vi "TAT_Start.vi"(8 "error In":errorcluster) -> (0 "error out":errorcluster)   [LabVIEW 2017]
uses:
  <vilib>/Utility/error.llb/DialogType.ctl
  Controls/Ass. Loop Control.ctl
  <vilib>/addons/database/Connection.llb/Conn ObjectReference.ctl
  227c0874-5cf7-40bb-b9d2-311cfb67fe7f.vi
  Global/Global 1.vi
  <vilib>/Instr/_visa.llb/VISA Configure Serial Port (Instr).vi
  <vilib>/addons/database/NI_Database_API.lvlib
  <vilib>/Utility/config.llb/NI_LVConfig.lvlib
panel:
  in  "MODEL SELECTION:-":string(combo)
  out "12 4":bool
  out "EOL AUTO CYCLE STATUS:-":bool
  out "12 3":bool
  out "12 2":bool
  out "12":bool
  out "PLC STATUS:-":bool
  out "array":string[](array[string])
  out "LEAK UNIT RESULT 2":bool caption="LEAK RESULT:-"
  out "LEAK ACTUAL VALUE 2":string
  out "LEAK MAX 2":string
  out "LEAK MIN 2":string
  out "LEAK UNIT RESULT":bool caption="LEAK RESULT:-"
  out "LEAK ACTUAL VALUE":string
  out "LEAK MAX":string
  out "LEAK MIN":string
  out "PREVIOUS BARCODE":string[](array[string])
  out "scanned":string
  out "Scanned Qyt":string
  out "PROJECT :-":string
  out "PACKAGE Qty":string
  out "TORISHI CODE:-":string
  out "PART No.:-":string
  in  "Stop":bool
  out "BARCODE STATION 2":string caption="BARCODE:-"
  out "RESULT STATION 1":bool caption="FINAL RESULT:-"
  out "USER:-":string
  out "PART NAME :-":string
  in  "ASS-Alarms":bool
  out "CYCLE STATUS STATION 1":string caption="CYCLE STATUS:-"
  out "DATE/TIME":string
  # "KAPSE SONS ROBOTICS\n& AUTOMATION"
  # "Nm"
  # "POKA-YOKE STATUS"
  # "LEAK TESTING PARAMETER"
  # "MIN"
  # "MAX"
  # "ACTUAL VALUE"
  # "RESULT"
  # "LEAK UNIT"
  # "LEAK PRESSURE"
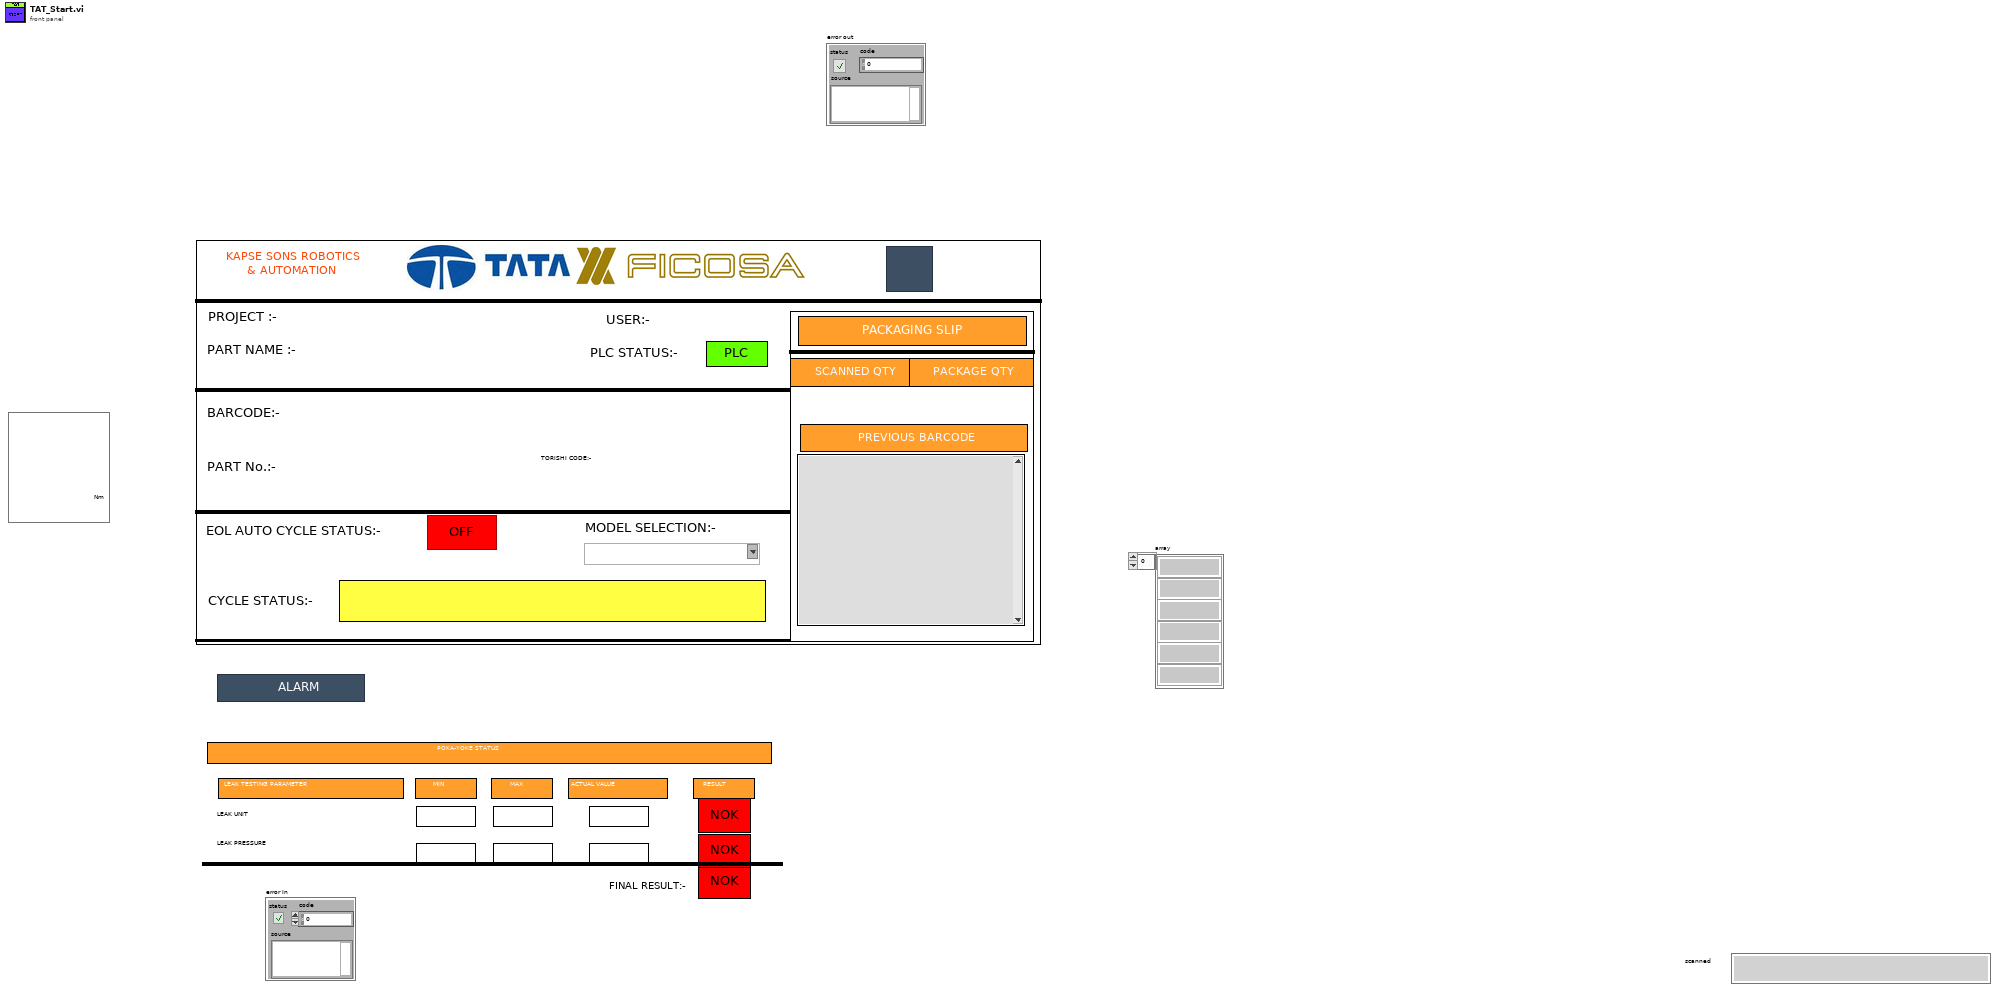
[diagram p1: front panel]
types:
  T1 = typedef "NI_Database_API.lvlib/Conn ObjectReference.ctl" = refnum<k1>
  T2 = cluster{"Varient number":u16, "Part name":string, "Barcode":string, "connection reference":T1, "Batch_Size":u16, "PART_NO":string, "TORISHI_CODE":string, "scanner com":refnum<visa-resource-name>, "Part Name List":string[], "Varient path":path, "Current Varient path":path, "Communication path":path, "PRN path":path, "printer":refnum<k5>, "Data_log_Path":path, "PREVIOUS Code":string[], "Printer IP add":string}
  T3 = typedef "Ass. Loop Control.ctl" = enum16{"Int2", "Package_Qty_Count", "GENERATE_QR_PRNT", "Cluster_update", "Waiting_for_scan", "barcode CHECK", "Int", "SaveReport ", "Barcode Print", "Start Cycle", "Wait", "Cycle End", "Stop"}
  T4 = typedef "DialogType.ctl" = u16
  T5 = enum32{"invalid app kind", "Development System", "Run Time System", "Student Edition", "Embedded LabVIEW", "Evaluation", "Custom"}
  T6 = typedef "NI_LVConfig.lvlib/Config Data RefNum.ctl" = refnum<k1>
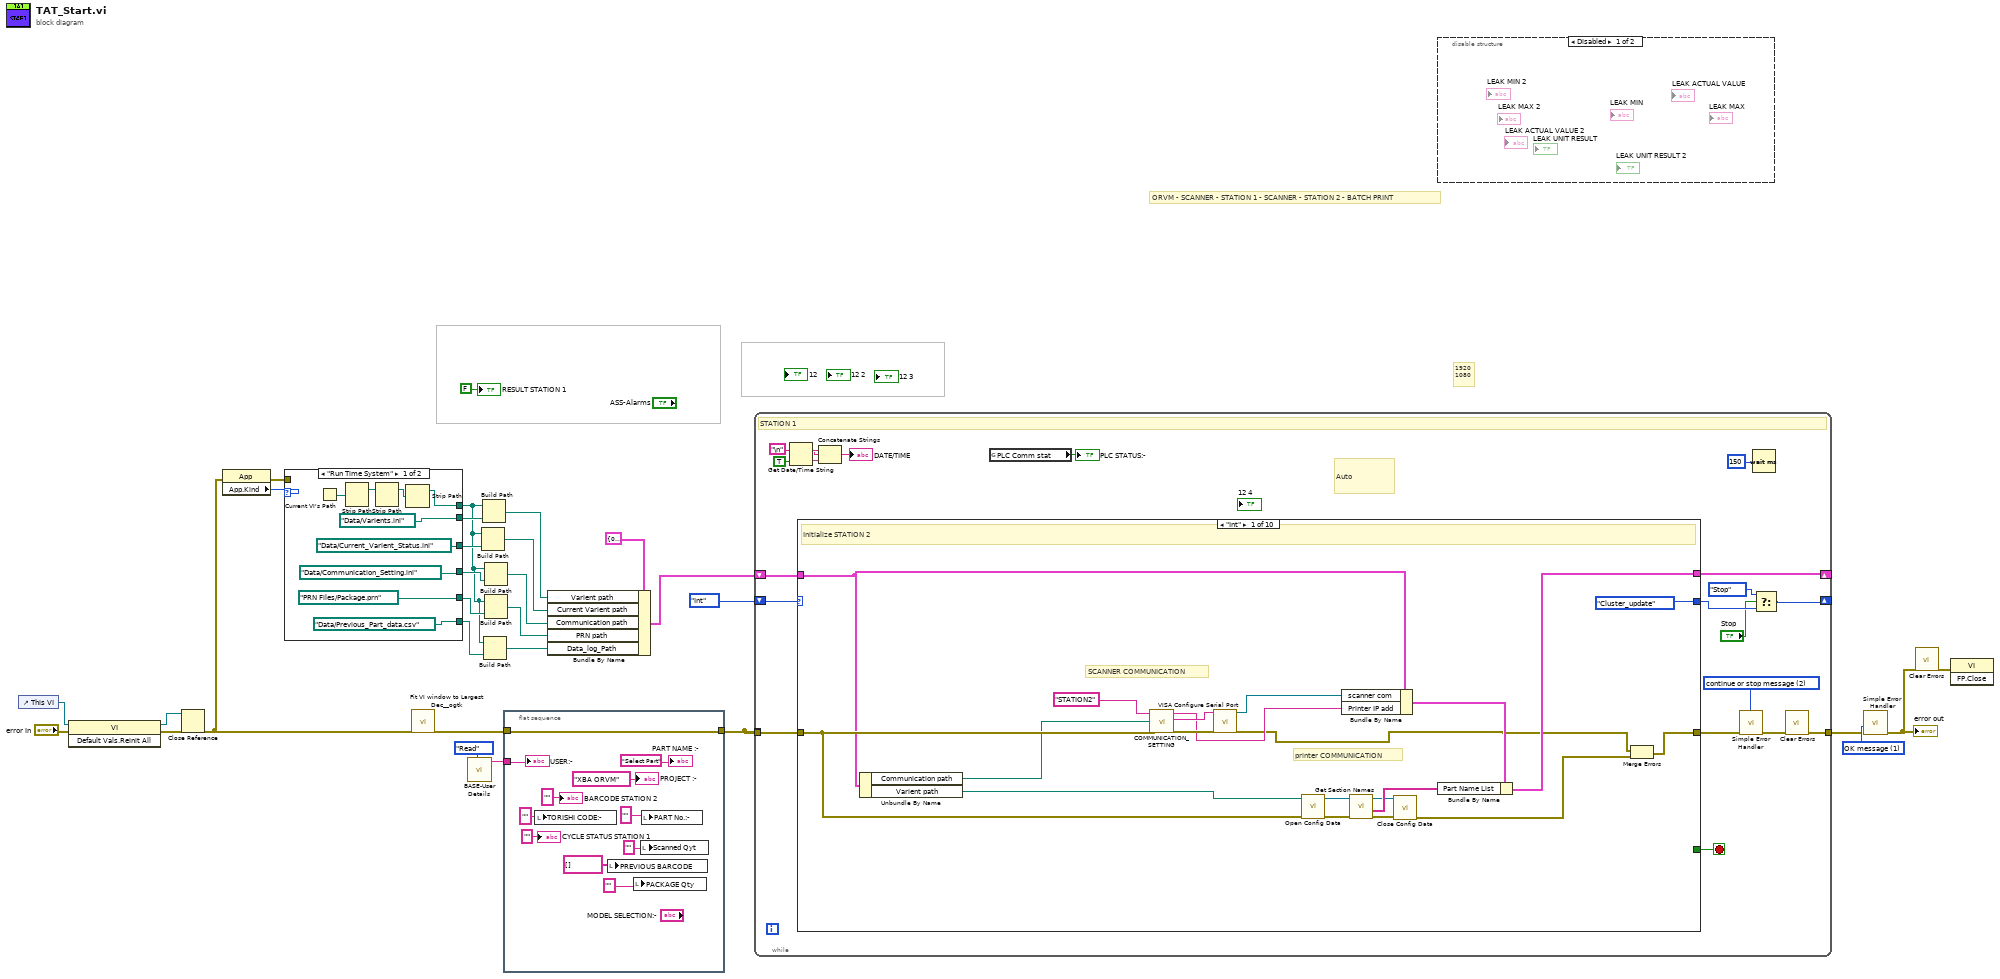
[diagram p0: block diagram]
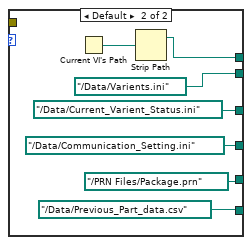
[diagram p2: hidden frame]
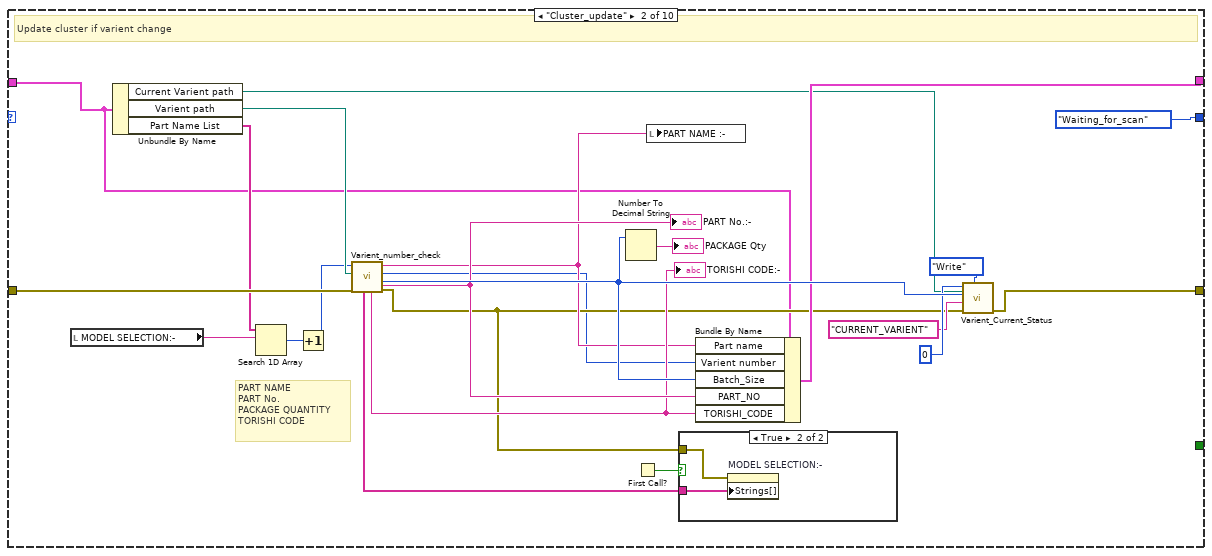
[diagram p4: hidden frame]
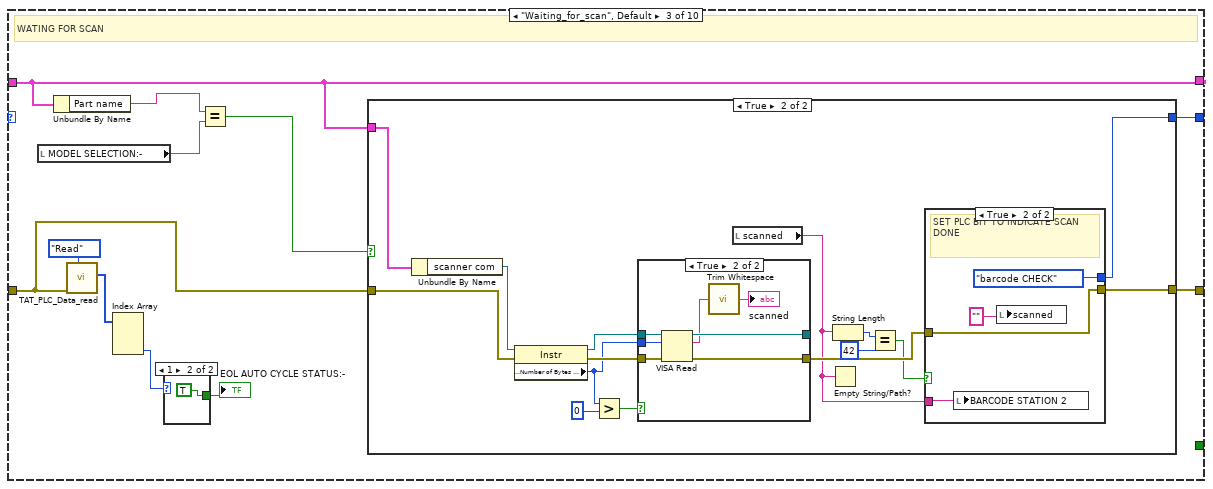
[diagram p6: hidden frame]
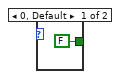
[diagram p7: hidden frame]
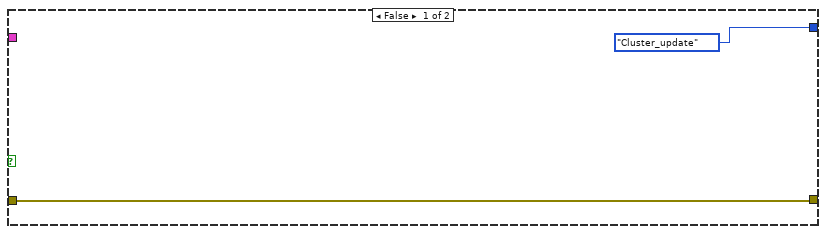
[diagram p8: hidden frame]
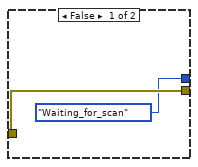
[diagram p10: hidden frame]
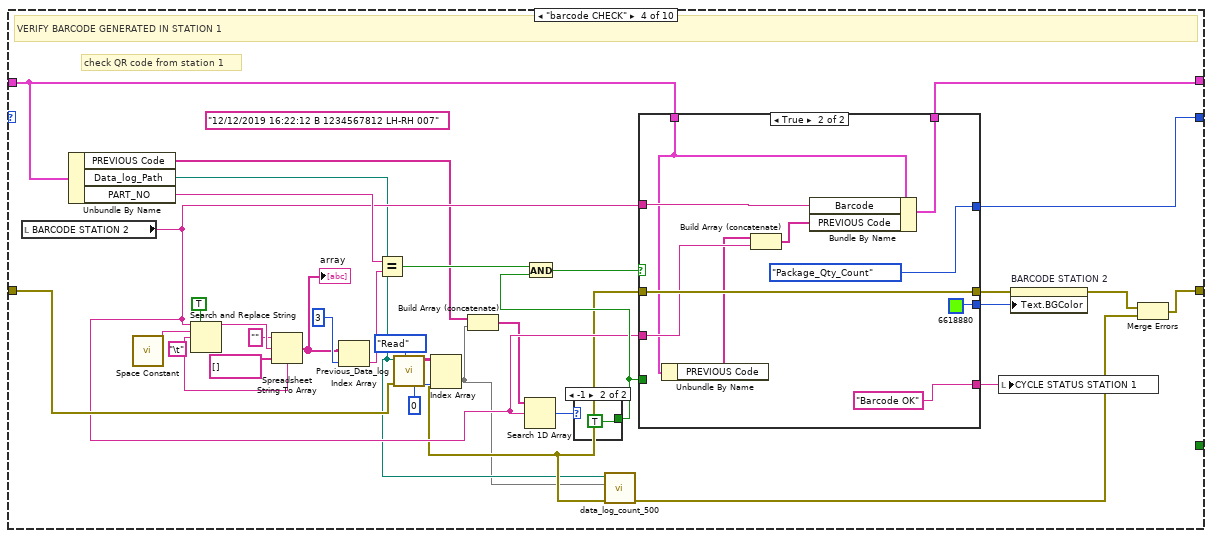
[diagram p11: hidden frame]
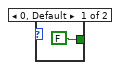
[diagram p12: hidden frame]
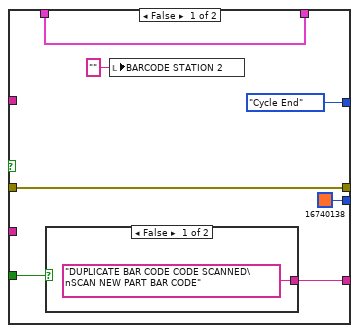
[diagram p13: hidden frame]
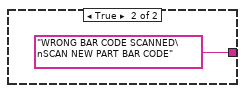
[diagram p14: hidden frame]
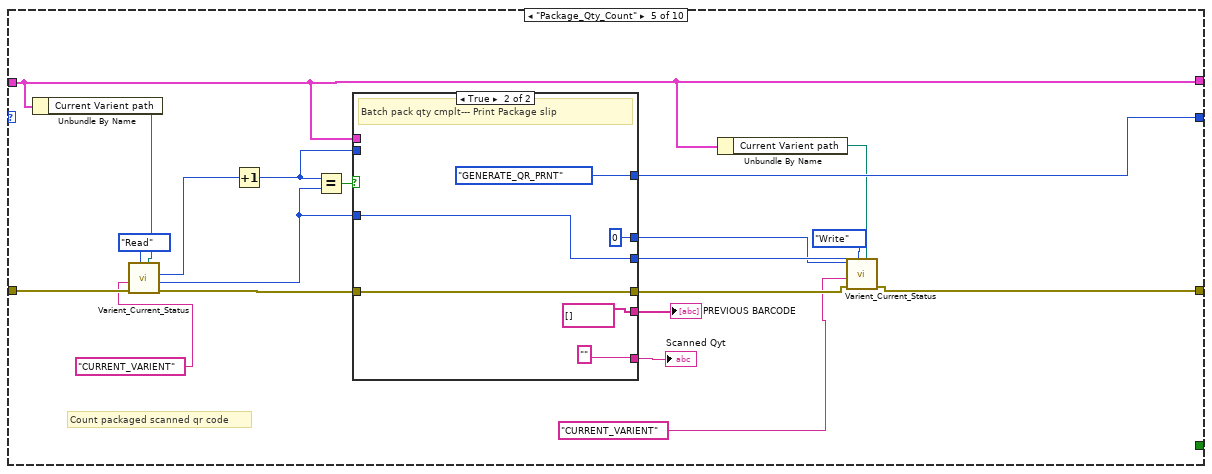
[diagram p15: hidden frame]
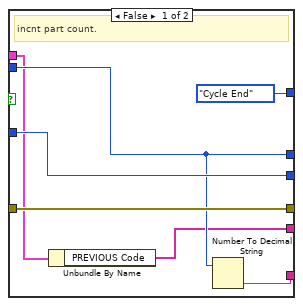
[diagram p16: hidden frame]
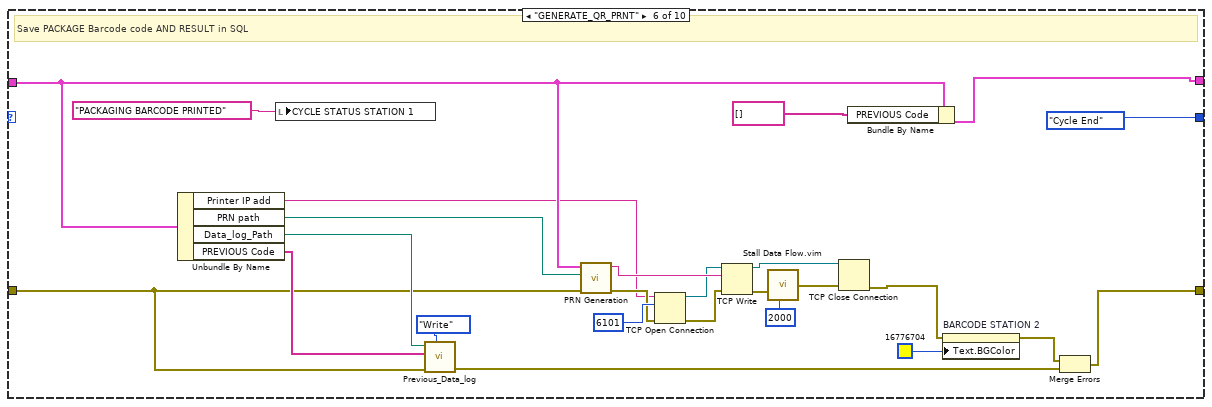
[diagram p17: hidden frame]
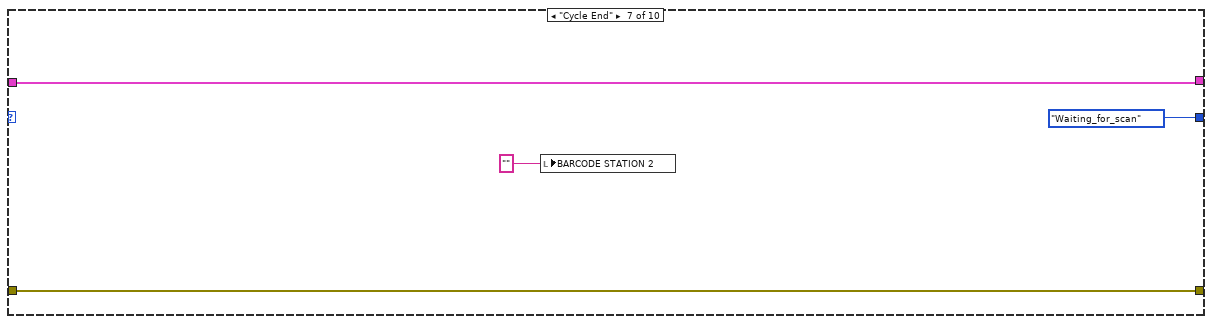
[diagram p18: hidden frame]
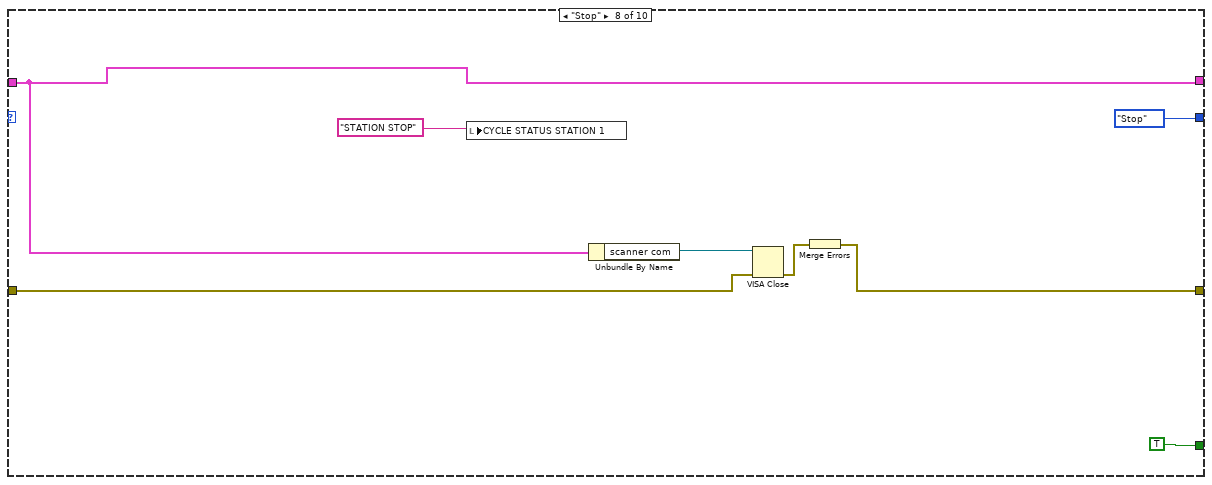
[diagram p19: hidden frame]
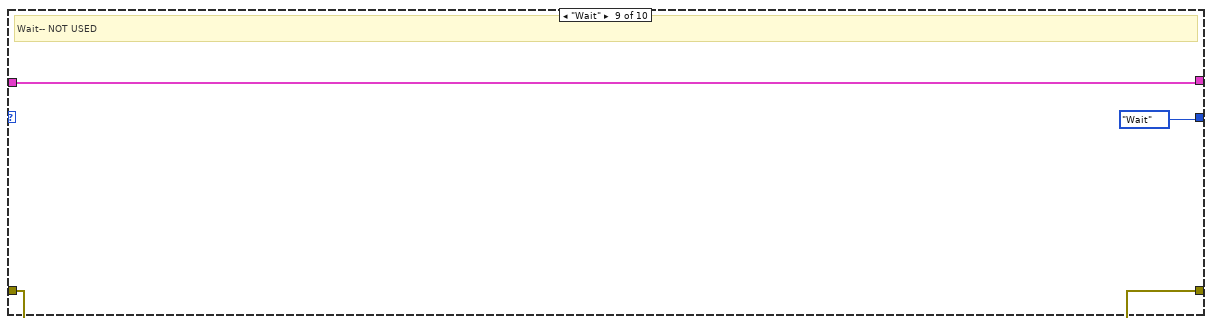
[diagram p20: hidden frame]
diagram:
  w20 = T4 1 items=["no dialog", "OK message", "continue or stop message", "OK message + warnings", "continue/stop + warnings"] ("type of dialog (OK msg:1)")
  # "1920\n1080"
  # "ORVM - SCANNER - STATION 1 - SCANNER - STATION 2 - BATCH PRINT"
  n1 = control-ref of="This VI"() -> (w30:refnum<vi>)
  n2 = invoke class="VI" method="Default Vals.Reinit All"(reference=w30, error in="error In") -> (reference out=w27:refnum<vi>, error out=w28:errorcluster)  [unwired: 1 in, 1 out]
  n3 = Close Reference(reference=w27, error in (no error)=w28) -> (error out=w4:errorcluster)
  n4 = property class="App"(error in=w4) -> (error out=w7:errorcluster, "App.Kind"=w16:T5)  [unwired: 1 in, 1 out]
  n5 = case shown="\"Run Time System\"" w16 {
    tunnel: [path "Data/Varients.ini" ("path") path "../Data/Varients.ini" ("path")] -> w15
    tunnel: [w35 w44] -> w5
    tunnel: [path "Data/Current_Varient_Status.ini" ("path") path "../Data/Current_Varient_Status.ini" ("path")] -> w12
    tunnel: [path "Data/Communication_Setting.ini" ("path") path "../Data/Communication_Setting.ini" ("path")] -> w11
    tunnel: [path "PRN Files/Package.prn" ("path") path "../PRN Files/Package.prn" ("path")] -> w9
    tunnel: w7 -> [_ _]
    tunnel: [path "Data/Previous_Part_data.csv" ("path") path "../Data/Previous_Part_data.csv" ("path")] -> w1
    frame "Run Time System" {
      n6 = Current VI's Path() -> (path=w38:path)
      n7 = Strip Path(path=w38) -> (stripped path=w37:path)  [unwired: 1 out]
      n8 = Strip Path(path=w37) -> (stripped path=w36:path)  [unwired: 1 out]
      n9 = Strip Path(path=w36) -> (stripped path=w35:path)  [unwired: 1 out]
    }
    frame Default {
      n10 = Current VI's Path() -> (path=w45:path)
      n11 = Strip Path(path=w45) -> (stripped path=w44:path)  [unwired: 1 out]
    }
  }
  n12 = call <userlib>:"Fit VI window to Largest Dec__ogtk.vi"("error in (no error)"=w4) -> ("error out"=w26:errorcluster)  [unwired: 5 in, 1 out]
  n13 = call "BASE-User Details.vi"("Enum"=enum16{"Read", "Write"}."Read") -> ("User Name Out"=w21:string)  [unwired: 9 in, 1 out]
  n14 = Build Path(base path=w5, name or relative path=w12) -> (appended path=w13:path)
  n15 = Build Path(base path=w5, name or relative path=w15) -> (appended path=w14:path)
  n16 = Build Path(base path=w5, name or relative path=w1) -> (appended path=w6:path)
  n17 = Build Path(base path=w5, name or relative path=w11) -> (appended path=w10:path)
  n18 = Build Path(base path=w5, name or relative path=w9) -> (appended path=w8:path)
  n19 = flat-sequence {
    tunnel: [w57] -> w18
    tunnel: w26 -> [w57]
    tunnel: w21 -> [w56]
    frame #0 {
      n20 = local write "TORISHI CODE:-"("") -> ()
      n21 = local write "PREVIOUS BARCODE"(string[] []) -> ()
      n22 = local write "PACKAGE Qty"("") -> ()
      n23 = local write "Scanned Qyt"("") -> ()
      n24 = local write "PART No.:-"("") -> ()
      "USER:-" <- w56
      "PART NAME :-" <- "Select Part"
      "PROJECT :-" <- "XBA ORVM" ("PROJECT")
      "BARCODE STATION 2" <- ""
      "CYCLE STATUS STATION 1" <- ""
    }
  }
  n25 = Bundle By Name(cluster=T2 {"Varient number"=0, "Part name"="", "Barcode"="", "connection reference"=refnum, "Batch_Size"=0, "PART_NO"="", "TORISHI_CODE"="", "scanner com"="", "Part Name List"=[], "Varient path"=path "", "Current Varient path"=path "", "Communication path"=path "", "PRN path"=path "", "printer"=refnum, "Data_log_Path"=path "", "PREVIOUS Code"=[], "Printer IP add"=""}, "Varient path"=w14, "Current Varient path"=w13, "Communication path"=w10, "PRN path"=w8, "Data_log_Path"=w6) -> (w2:T2)
  n26 = while {
    tunnel: w18 -> [_]
    shift-right: [w66] -> _
    shift-left: Ass._Loop_Control."Int" ("Enum") -> [w71]
    tunnel: w18 -> [w70]
    shift-right: [w68] -> _
    shift-left: w2 -> [w69]
    tunnel: [w59] -> w17
    stop <- w58 stop-if-true
    w63 = T4 2 items=["no dialog", "OK message", "continue or stop message", "OK message + warnings", "continue/stop + warnings"] ("type of dialog (OK msg:1)")
    # "Auto"
    # "STATION 1"
    n27 = Get Date/Time String(want seconds? (F)=TRUE) -> (date string=w75:string, time string=w74:string)  [unwired: 2 in]
    n28 = case shown="\"Int\"" w71 {
      tunnel: [Ass._Loop_Control."Cluster_update" ("Enum") Ass._Loop_Control."Waiting_for_scan" ("Enum") w132 w176 w230 Ass._Loop_Control."Cycle End" ("Enum") Ass._Loop_Control."Waiting_for_scan" ("Enum") Ass._Loop_Control."Stop" ("Enum") Ass._Loop_Control."Wait" ("Enum") Ass._Loop_Control."Wait" ("Enum")] -> w65
      tunnel: [w84 w112 w129 w198 w222 w274 w282 w287 w294 w295] -> w68
      tunnel: [w83 w113 w133 w173 w235 w266 w280 w288 w292 w296] -> w62
      tunnel: w70 -> [w93 w107 w123 w180 w241 w268 w280 w285 w292 w296]
      tunnel: w69 -> [w92 w98 w129 w199 w222 w263 w282 w287 w294 w295]
      tunnel: [_ _ _ _ _ _ _ TRUE _ _] -> w58
      frame "Int" {
        # "printer COMMUNICATION"
        # "SCANNER COMMUNICATION"
        # "Initialize STATION 2"
        n29 = Unbundle By Name(w92) -> ("Communication path"=w81:path, "Varient path"=w82:path)
        n30 = call "COMMUNICATION_SETTING.vi"("communication path"=w81, "error in"=w93, "STATION"="STATION2") -> ("error out"=w96:errorcluster, "SCAN_COM"=w94:string, "PRINT_COM"=w80:string)  [unwired: 6 in]
        n31 = call-poly "VISA Configure Serial Port"("VISA resource name"=w94, "error in (no error)"=w96) -> ("VISA resource name out"=w78:refnum<visa-resource-name>, "error out"=w79:errorcluster)  [unwired: 12 in]
        n32 = call <vilib>:"Open Config Data.vi"("error in (no error)"=w93, "configuration file path"=w82) -> ("error out"=w89:errorcluster, "refnum"=w90:T6)  [unwired: 7 in, 1 out]
        n33 = Bundle By Name(cluster=w92, "scanner com"=w78, "Printer IP add"=w80) -> (w85:T2)
        n34 = call <vilib>:"Get Section Names.vi"("error in (no error)"=w89, "refnum"=w90) -> ("error out"=w88:errorcluster, "section names"=w91:string[], "refnum out"=w87:T6)  [unwired: 7 in]
        n35 = call <vilib>:"Close Config Data.vi"("error in (no error)"=w88, "refnum"=w87) -> ("error out"=w86:errorcluster)  [unwired: 8 in, 1 out]
        n36 = Bundle By Name(cluster=w85, "Part Name List"=w91) -> (w84:T2)
        n37 = Merge Errors(w79, w86) -> (w83:errorcluster)
      }
      frame "Cluster_update" {
        # "PART NAME\nPART No.\nPACKAGE QUANTITY\nTORISHI CODE"
        # "Update cluster if varient change"
        n38 = local read "MODEL SELECTION:-"() -> (w101:string)
        n39 = Unbundle By Name(w98) -> ("Current Varient path"=w108:path, "Varient path"=w109:path, "Part Name List"=w102:string[])
        n40 = Search 1D Array(1D array=w102, element=w101) -> (index of element=w103:i32)  [unwired: 1 in]
        n41 = Increment(x=w103) -> (x+1=w100:i32)
        n42 = call "Varient_number_check.vi"("error in"=w107, "Varient path"=w109, "Varient No."=w100) -> ("error out"=w104:errorcluster, "Batch Size"=w120:i32, "Varient Number"=w99:i32, "Part Name"=w116:string, "PART_NO"=w119:string, "TORISHI_CODE"=w118:string, "MODEL LIST"=w105:string[])  [unwired: 2 in]
        "PART No.:-" <- w119
        "TORISHI CODE:-" <- w118
        n43 = Number To Decimal String(number=w120) -> (decimal integer string=→"PACKAGE Qty":string)  [unwired: 1 in]
        n44 = First Call?() -> (First Call?: T/F=w106:bool)
        n45 = local write "PART NAME :-"(w116) -> ()
        n46 = case shown="True" w106 {
          tunnel: w105 -> [_ w122]
          tunnel: w104 -> [_ w121]
          frame False {
          }
          frame True {
            n47 = property on="MODEL SELECTION:-" class="CmbBox"(error in=w121, "Strings[]"=w122) -> ()  [unwired: 1 in, 2 out]
          }
        }
        n48 = Bundle By Name(cluster=w98, "Part name"=w116, "Varient number"=w99, "Batch_Size"=w120, "PART_NO"=w119, "TORISHI_CODE"=w118) -> (w112:T2)
        n49 = call "Varient_Current_Status.vi"("Currenrt Varient path"=w108, "Enum"=enum16{"Write", "Read"}."Write", "error in"=w104, "AUTO/MANUAL"="CURRENT_VARIENT", "Batch Size"=w120, "Varient count"=0) -> ("error out"=w113:errorcluster)  [unwired: 3 in, 2 out]
      }
      frame "Waiting_for_scan", Default {
        # "WATING FOR SCAN"
        n50 = local read "MODEL SELECTION:-"() -> (w126:string)
        n51 = Unbundle By Name(w129) -> ("Part name"=w125:string)
        n52 = call "TAT_PLC_Data_read.vi"("Enum"=enum16{"Read", "Write"}."Read", "error in (no error)"=w123) -> ("Array 2"=w130:u16[])  [unwired: 8 in, 1 out]
        n53 = Index Array(array=w130) -> (element #3=w128:u16)  [unwired: 3 in, 2 out]
        n54 = case shown="1" w128 {
          tunnel: [FALSE TRUE] -> w127
          frame 0, Default {
          }
          frame 1 {
          }
        }
        "EOL AUTO CYCLE STATUS:-" <- w127
        n55 = Equal?(x=w125, y=w126) -> (x = y?=w124:bool)
        n56 = case shown="True" w124 {
          tunnel: [w137 w149] -> w133
          tunnel: [Ass._Loop_Control."Cluster_update" ("Enum") w148] -> w132
          tunnel: w123 -> [w137 w139]
          tunnel: w129 -> [_ w138]
          frame False {
          }
          frame True {
            n57 = Unbundle By Name(w138) -> ("scanner com"=w147:refnum<visa-resource-name>)
            n58 = property class="Instr"(reference=w147, error in=w139) -> (reference out=w152:refnum<visa-resource-name>, error out=w151:errorcluster, "Serial Settings:Number of Bytes at Serial Port"=w146:u32)
            n59 = Greater?(x=w146, y=u32 0) -> (0:w145:bool)
            n60 = case shown="True" w145 {
              tunnel: w152 -> [w154 w161]
              tunnel: w151 -> [w153 w160]
              tunnel: w146 -> [_ w159]
              tunnel: [w154 w158] -> _
              tunnel: [w153 w155] -> w150
              frame False {
              }
              frame True {
                n61 = VISA Read(VISA resource name=w161, byte count=w159, error in (no error)=w160) -> (VISA resource name out=w158:refnum<visa-resource-name>, read buffer=w156:string, error out=w155:errorcluster)  [unwired: 1 out]
                n62 = call <vilib>:"Trim Whitespace.vi"("string"=w156) -> ("trimmed string"=→"scanned":string)  [unwired: 1 in]
              }
            }
            n63 = local read "scanned"() -> (w143:string)
            n64 = Empty String/Path?(string/path=w143) -> ()  [unwired: 1 out]
            n65 = String Length(string=w143) -> (length=w142:i32)
            n66 = Equal?(x=w142, y=42) -> (x = y?=w140:bool)
            n67 = case shown="True" w140 {
              tunnel: w150 -> [w163 w167]
              tunnel: [w163 w167] -> w149
              tunnel: w143 -> [_ w166]
              tunnel: [Ass._Loop_Control."Waiting_for_scan" ("Enum") Ass._Loop_Control."barcode CHECK" ("Enum")] -> w148
              frame False {
              }
              frame True {
                # "SET PLC BIT TO INDICATE SCAN DONE"
                n68 = local write "BARCODE STATION 2"(w166) -> ()
                n69 = local write "scanned"("") -> ()
              }
            }
          }
        }
      }
      frame "barcode CHECK" {
        w194 = "\t"
        (unwired) "12/12/2019 16:22:12 B 1234567812 LH-RH 007" ("string")
        # "check QR code from station 1"
        # "VERIFY BARCODE GENERATED IN STATION 1"
        n70 = local read "BARCODE STATION 2"() -> (w177:string)
        n71 = Unbundle By Name(w199) -> ("PREVIOUS Code"=w170:string[], "Data_log_Path"=w171:path, "PART_NO"=w190:string)
        n72 = call <vilib>:"Space Constant.vi"() -> ("String"=w197:string)
        n73 = Search and Replace String(replace all?=TRUE ("replace all? (F)"), input string=w177, search string=w197, replace string=w194) -> (result string=w195:string)  [unwired: 4 in, 3 out]
        n74 = Spreadsheet String To Array(delimiter (Tab)=w194, format string="", spreadsheet string=w195, array type (2D Dbl)=string[] []) -> (array=w186:string[])
        "array" <- w186
        n75 = Index Array(array=w186, index=3) -> (element=w189:string)
        n76 = Equal?(x=w190, y=w189) -> (x = y?=w188:bool)
        n77 = call "Previous_Data_log.vi"(7:enum16{"Write", "Read"}."Read", "error in (no error)"=w180, "file path (dialog if empty)"=w171) -> ("error out"=w175:errorcluster, "all rows"=w183:string[][])  [unwired: 7 in]
        n78 = Index Array(array=w183, index (col)=0 ("disabled index (col)")) -> (element=w169:string[])  [unwired: 1 in]
        n79 = Build Array (concatenate)(w170, w169) -> (w168:string[])
        n80 = Search 1D Array(1D array=w168, element=w177) -> (index of element=w184:i32)  [unwired: 1 in]
        n81 = case shown="-1" w184 {
          tunnel: [FALSE TRUE] -> w179
          frame 0, Default {
          }
          frame -1 {
          }
        }
        n82 = And(x=w188, y=w179) -> (x .and. y?=w187:bool)
        n83 = call "data_log_count_500.vi"("error in (no error)"=w175, "All data"=w169, "file path (dialog if empty)"=w171) -> ("error out"=w172:errorcluster)  [unwired: 8 in]
        n84 = case shown="True" w187 {
          tunnel: [w209 "Barcode OK" ("Cycle Status")] -> w200
          tunnel: w199 -> [w208 w214]
          tunnel: [w208 w220] -> w198
          tunnel: w177 -> [_ w219]
          tunnel: [u32 16740138 u32 6618880] -> w185
          tunnel: w179 -> [w203 _]
          tunnel: w175 -> [w206 w217]
          tunnel: [w206 w217] -> w178
          tunnel: w177 -> [_ w215]
          tunnel: [Ass._Loop_Control."Cycle End" ("Enum") Ass._Loop_Control."Package_Qty_Count" ("Enum")] -> w176
          frame False {
            n85 = case shown="False" w203 {
              tunnel: ["DUPLICATE BAR CODE CODE SCANNED\nSCAN NEW PART BAR CODE" ("Cycle Status") "WRONG BAR CODE SCANNED\nSCAN NEW PART BAR CODE" ("Cycle Status")] -> w209
              frame False {
              }
              frame True {
              }
            }
            n86 = local write "BARCODE STATION 2"("" ("BARCODE STATION 2")) -> ()
          }
          frame True {
            n87 = Unbundle By Name(w214) -> ("PREVIOUS Code"=w213:string[])
            n88 = Build Array (concatenate)(w213, w215) -> (w216:string[])
            n89 = Bundle By Name(cluster=w214, "Barcode"=w219, "PREVIOUS Code"=w216) -> (w220:T2)
          }
        }
        n90 = local write "CYCLE STATUS STATION 1"(w200) -> ()
        n91 = property on="BARCODE STATION 2" class="Str"(error in=w178, "Text.BGColor"=w185) -> (error out=w174:errorcluster)  [unwired: 1 in, 1 out]
        n92 = Merge Errors(w174, w172) -> (w173:errorcluster)
      }
      frame "Package_Qty_Count" {
        # "Count packaged scanned qr code"
        n93 = Unbundle By Name(w222) -> ("Current Varient path"=w226:path)
        n94 = call "Varient_Current_Status.vi"("Currenrt Varient path"=w226, "Enum"=enum16{"Write", "Read"}."Read", "error in"=w241, "AUTO/MANUAL"="CURRENT_VARIENT") -> ("error out"=w239:errorcluster, "Batch Size"=w233:i32, "Varient Count"=w238:i32)  [unwired: 5 in]
        n95 = Increment(x=w238) -> (x+1=w225:i32)
        n96 = Equal?(x=w225, y=w233) -> (x = y?=w237:bool)
        n97 = case shown="True" w237 {
          tunnel: [w248 w254] -> w234
          tunnel: w239 -> [w248 w254]
          tunnel: w225 -> [w244 _]
          tunnel: w233 -> [w247 w253]
          tunnel: [w247 w253] -> w232
          tunnel: [w244 0] -> w231
          tunnel: [Ass._Loop_Control."Cycle End" ("Enum") Ass._Loop_Control."GENERATE_QR_PRNT" ("Enum")] -> w230
          tunnel: [w242 string[] [] ("PREVIOUS BARCODE")] -> w224
          tunnel: [w245 ""] -> w223
          tunnel: w222 -> [w243 _]
          frame False {
            # "incnt part count."
            n98 = Unbundle By Name(w243) -> ("PREVIOUS Code"=w242:string[])
            n99 = Number To Decimal String(number=w244) -> (decimal integer string=w245:string)  [unwired: 1 in]
          }
          frame True {
            # "Batch pack qty cmplt--- Print Package slip"
          }
        }
        "PREVIOUS BARCODE" <- w224
        "Scanned Qyt" <- w223
        n100 = Unbundle By Name(w222) -> ("Current Varient path"=w227:path)
        n101 = call "Varient_Current_Status.vi"("Currenrt Varient path"=w227, "Enum"=enum16{"Write", "Read"}."Write", "error in"=w234, "AUTO/MANUAL"="CURRENT_VARIENT", "Batch Size"=w232, "Varient count"=w231) -> ("error out"=w235:errorcluster)  [unwired: 3 in, 2 out]
      }
      frame "GENERATE_QR_PRNT" {
        # "Save PACKAGE Barcode code AND RESULT in SQL"
        n102 = Unbundle By Name(w263) -> ("Printer IP add"=w255:string, "PRN path"=w273:path, "Data_log_Path"=w270:path, "PREVIOUS Code"=w269:string[])
        n103 = local write "CYCLE STATUS STATION 1"("PACKAGING BARCODE PRINTED" ("Cycle Status")) -> ()
        n104 = call "Previous_Data_log.vi"(7:enum16{"Write", "Read"}."Write", "error in (no error)"=w268, "Data IN"=w269, "file path (dialog if empty)"=w270) -> ("error out"=w265:errorcluster)  [unwired: 6 in, 1 out]
        n105 = call "PRN Generation.vi"("error in (no error)"=w268, "PRN path"=w273, "Cluster"=w263) -> ("error out"=w261:errorcluster, "PRN to Print"=w277:string)  [unwired: 7 in]
        n106 = TCP Open Connection(address=w255, remote port or service name=u16 6101, error in (no error)=w261) -> (connection ID=w259:refnum<k5>, error out=w260:errorcluster)  [unwired: 2 in]
        n107 = TCP Write(connection ID=w259, data in=w277, error in (no error)=w260) -> (connection ID out=w256:refnum<k5>, error out=w264:errorcluster)  [unwired: 1 in, 1 out]
        n108 = call "Stall Data Flow.vim"("value in"=w264, "milliseconds to wait"=u32 2000) -> ("value out"=w258:errorcluster)  [unwired: 1 out]
        n109 = TCP Close Connection(connection ID=w256, error in (no error)=w258) -> (error out=w257:errorcluster)  [unwired: 1 in, 1 out]
        n110 = Bundle By Name(cluster=w263, "PREVIOUS Code"=string[] []) -> (w274:T2)
        n111 = property on="BARCODE STATION 2" class="Str"(error in=w257, "Text.BGColor"=u32 16776704) -> (error out=w267:errorcluster)  [unwired: 1 in, 1 out]
        n112 = Merge Errors(w267, w265) -> (w266:errorcluster)
      }
      frame "Cycle End" {
        n113 = local write "BARCODE STATION 2"("" ("BARCODE STATION 2")) -> ()
      }
      frame "Stop" {
        n114 = local write "CYCLE STATUS STATION 1"("STATION STOP" ("Cycle Status")) -> ()
        n115 = Unbundle By Name(w287) -> ("scanner com"=w286:refnum<visa-resource-name>)
        n116 = VISA Close(VISA resource name=w286, error in (no error)=w285) -> (error out=w289:errorcluster)
        n117 = Merge Errors(w289) -> (w288:errorcluster)
      }
      frame "Wait" {
        # "Wait-- NOT USED"
      }
      frame "Start Cycle" {
        n118 = local write "CYCLE STATUS STATION 1"("Cycle started" ("Cycle Status")) -> ()
      }
    }
    n119 = Concatenate Strings(w75, "\n", w74) -> (→"DATE/TIME":string)
    n120 = global read "Global 1.vi" "PLC Comm stat"() -> (→"PLC STATUS:-":bool)
    n121 = call <vilib>:"Simple Error Handler.vi"("type of dialog (OK msg:1)"=w63, "error in (no error)"=w62) -> ("error out"=w60:errorcluster)  [unwired: 3 in, 4 out]
    n122 = Wait (ms)(milliseconds to wait=u32 150) -> ()  [unwired: 1 out]
    n123 = Select(t=Ass._Loop_Control."Stop" ("Enum"), s="Stop", f=w65) -> (s? t:f=w66:T3)
    n124 = call <vilib>:"Clear Errors.vi"("error in (no error)"=w60) -> ("error out"=w59:errorcluster)  [unwired: 5 in, 1 out]
  }
  n125 = disable-structure shown="Disabled" {
    frame Disabled {
    }
    frame Enabled {
    }
  }
  n126 = call <vilib>:"Simple Error Handler.vi"("type of dialog (OK msg:1)"=w20, "error in (no error)"=w17) -> ("error out"=w24:errorcluster)  [unwired: 3 in, 4 out]
  "error out" <- w24
  n127 = call <vilib>:"Clear Errors.vi"("error in (no error)"=w24) -> ("error out"=w23:errorcluster)  [unwired: 5 in, 1 out]
  n128 = invoke class="VI" method="FP.Close"(error in=w23) -> ()  [unwired: 2 in, 3 out]
  "RESULT STATION 1" <- FALSE ("want seconds? (F)")
